vi "Xml_Load_Timing_Table.vi"(7 "Version String":string, 8 "error in (no error)":errorcluster, 10 "XML Path":path=path "D:/TEST.xml", 11 "Refnum Clust":refnum<vi>) -> (0 "error out":errorcluster)   [LabVIEW 2018]
uses:
  controls/TIMING_Table.ctl
  controls/TIMING_Mandatory_Items.ctl
  controls/TIMING_Optional_Items.ctl
panel:
  in  "TIMING Table":T1={"Mandatory Items"={"Script Name"="", "GINI Time Period"=100.0, "HSDIO Delay"=60.0, "Shutter Duration before"=50.0, "Shutter Duration after"=50.0, "Filter Tau"=2.0, "Trapping Delay"=600.0, "Trapping Duration"=300.0, "Emtyping Duration"=1000.0}, "Optional Items"={"Eject"=0, "Acq"=0, "Excit"=0, "Gas"=0, "Laser"=0, "Lamp"=0}, "Times Table"=[["Excit1", "name", "Swift", "0.5", "1200", "70", "150", "550", "0", "0", "0"]]} {"Optional Items"."Laser" min=0 max=3; "Optional Items"."Gas" min=0 max=5; "Mandatory Items"."GINI Time Period" min=100000.0 max=1000000.0 format="%#_7g"; "Mandatory Items"."Shutter Duration after" min=2.0 max=100000.0; "Mandatory Items"."HSDIO Delay" min=60.0 max=100.0; "Mandatory Items"."Shutter Duration before" min=2.0 max=100000.0; "Mandatory Items"."Filter Tau" min=1000.0 max=2000.0; "Mandatory Items"."Trapping Delay" min=2.0; "Mandatory Items"."Emtyping Duration" min=2.0 format="%#_8g"; "Mandatory Items"."Trapping Duration" min=2.0}
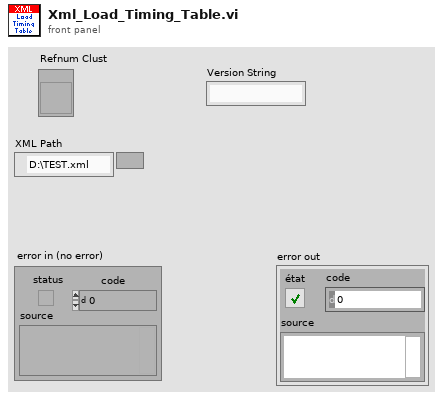
[diagram p1: front panel]
types:
  T1 = typedef "TIMING_Table.ctl" = cluster{"Mandatory Items":T2, "Optional Items":T3, "Times Table":string[][]}
  T2 = typedef "TIMING_Mandatory_Items.ctl" = cluster{"Script Name":string, "GINI Time Period":dbl, "HSDIO Delay":dbl, "Shutter Duration before":dbl, "Shutter Duration after":dbl, "Filter Tau":dbl, "Trapping Delay":dbl, "Trapping Duration":dbl, "Emtyping Duration":dbl}
  T3 = typedef "TIMING_Optional_Items.ctl" = cluster{"Eject":u32, "Acq":i32, "Excit":u32, "Gas":i32, "Laser":i32, "Lamp":i32}
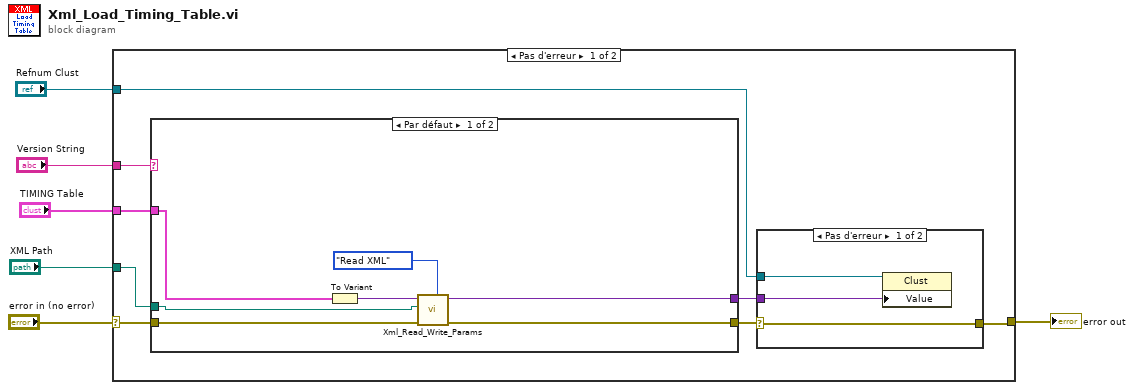
[diagram p0: block diagram]
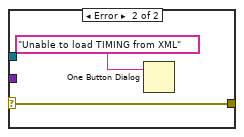
[diagram p2: hidden frame]
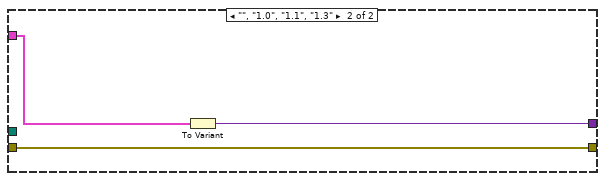
[diagram p3: hidden frame]
diagram:
  n1 = case shown="Pas d'erreur" "error in (no error)" {
    selector: "error in (no error)" -> [w14 w30]
    tunnel: [w9 w30] -> w6
    tunnel: "XML Path" -> [w13 _]
    tunnel: "Version String" -> [w12 _]
    tunnel: "Refnum Clust" -> [w7 _]
    tunnel: "TIMING Table" -> [w11 _]
    frame No Error {
      n2 = case shown="Par défaut" w12 {
        tunnel: w14 -> [w24 w28]
        tunnel: [w22 w28] -> w10
        tunnel: [w23 w29] -> w8
        tunnel: w13 -> [w21 _]
        tunnel: w11 -> [w20 w27]
        frame Default {
          n3 = To Variant(anything=w20) -> (Variant=w25:variant)
          n4 = call "Xml_Read_Write_Params.vi"("Variant"=w25, "XML Path"=w21, "error in (no error)"=w24, "Command"=enum16{"Read XML", "Set", "Get", "Write XML"}."Read XML") -> ("Variant Output"=w23:variant, "error out"=w22:errorcluster)  [unwired: 3 in, 1 out]
        }
        frame "", "1.0", "1.1", "1.3" {
          n5 = To Variant(anything=w27) -> (Variant=w29:variant)
        }
      }
      n6 = case shown="Pas d'erreur" w10 {
        selector: w10 -> [w16 w19]
        tunnel: w7 -> [w17 _]
        tunnel: [w16 w19] -> w9
        tunnel: w8 -> [w15 _]
        frame No Error {
          n7 = property class="Clust"(reference=w17, "Value"=w15) -> ()  [unwired: 1 in, 2 out]
        }
        frame Error {
          n8 = One Button Dialog(message="Unable to load TIMING from XML") -> ()  [unwired: 1 in, 1 out]
        }
      }
    }
    frame Error {
    }
  }
  "error out" <- w6
